vi "Swerve Data Normalize Velocity.vi"(10 "Calcualted Velocities Out":dbl[](array[numeric]), 11 "Swerve Data Out in":T1 {"Back Right"."Angle" scale format="%.3f"; "Back Right"."Velocity" scale=-1.0..1.0 scale format="%.1f"; "Back Left"."Angle" scale format="%.3f"; "Back Left"."Velocity" scale=-1.0..1.0 scale format="%.1f"; "Front Left"."Angle" scale format="%.3f"; "Front Left"."Velocity" scale=-1.0..1.0 scale format="%.1f"; "Front Right"."Angle" scale format="%.3f"; "Front Right"."Velocity" scale=-1.0..1.0 scale format="%.1f"}) -> (3 "Swerve Data Out out":T1 {"Back Right"."Angle" scale format="%.3f"; "Back Right"."Velocity" scale=-1.0..1.0 scale format="%.1f"; "Back Left"."Angle" scale format="%.3f"; "Back Left"."Velocity" scale=-1.0..1.0 scale format="%.1f"; "Front Left"."Angle" scale format="%.3f"; "Front Left"."Velocity" scale=-1.0..1.0 scale format="%.1f"; "Front Right"."Angle" scale format="%.3f"; "Front Right"."Velocity" scale=-1.0..1.0 scale format="%.1f"})   [LabVIEW 2023, in "TShirtWork-SwerveDrive_ACT_ts.lvlib"]
uses:
  TShirtWork-SwerveDrive_ACT_ts.lvlib
  Shared Code/TypeDefs/Cluster_Swerve 4 Steer and Velocity.ctl
  Shared Code/TypeDefs/Cluster_Module Velocity-Direction-Rotations.ctl
  Shared Code/TypeDefs/Level_Velocity plus-minus 1.ctl
  Shared Code/TypeDefs/Dial_Compase heading unit circle CCW positive.ctl
panel:
  # "\"Front\" of Robot"
  # "Right Hand Rule"
  # "X"
  # "+CCW"
  # "Y"
  # "(0,0)"
  # "\"Front\" of Robot"
  # "Right Hand Rule"
  # "X"
  # "+CCW"
  # "Y"
  # "(0,0)"
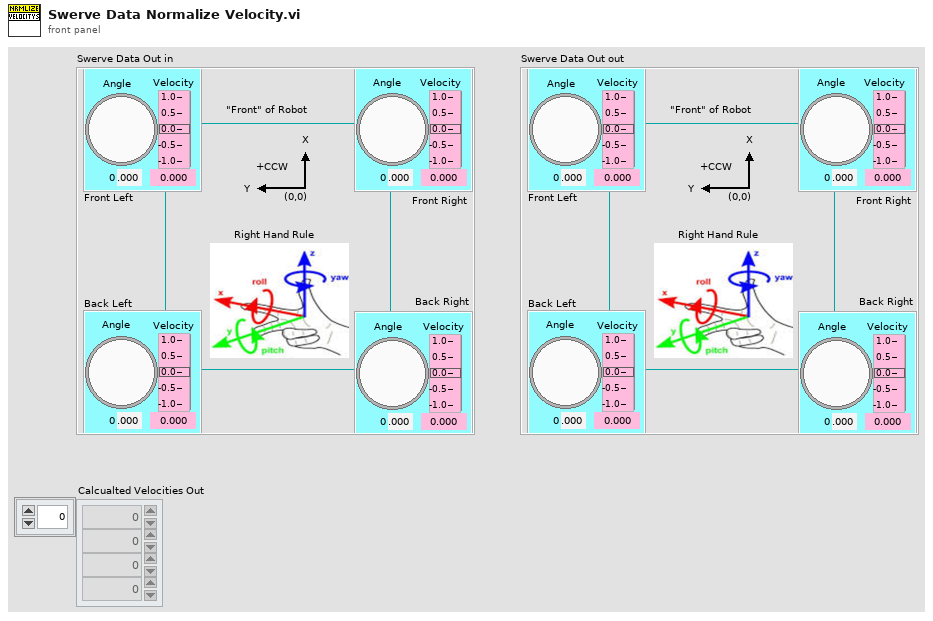
[diagram p1: front panel]
types:
  T1 = typedef "Cluster_Swerve 4 Steer and Velocity.ctl" = cluster{"Front Right":T2, "Front Left":T2, "Back Left":T2, "Back Right":T2}
  T2 = typedef "Cluster_Module Velocity-Direction-Rotations.ctl" = cluster{"Velocity":T3, "Angle":T4, "Rotations Count":dbl}
  T3 = typedef "Level_Velocity plus-minus 1.ctl" = dbl
  T4 = typedef "Dial_Compase heading unit circle CCW positive.ctl" = dbl
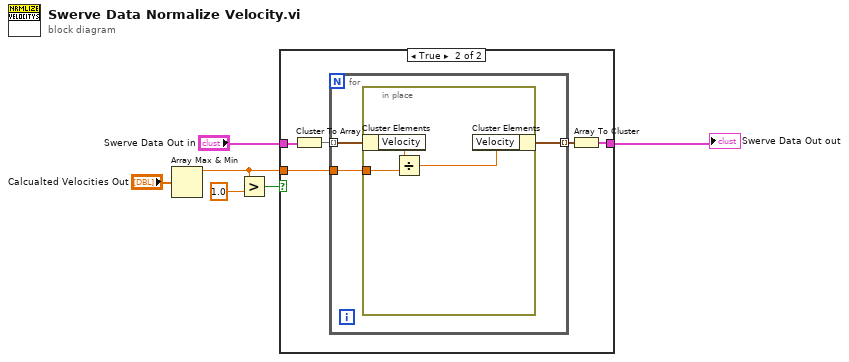
[diagram p0: block diagram]
diagram:
  n1 = Array Max & Min(array="Calcualted Velocities Out") -> (max value=w3:dbl)  [unwired: 3 out]
  n2 = Greater?(x=w3, y=1.0) -> (0:w2:bool)
  n3 = case shown="True" w2 {
    tunnel: "Swerve Data Out in" -> [w7 w12]
    tunnel: [w7 w9] -> w6
    tunnel: w3 -> [_ w8]
    frame False {
    }
    frame True {
      n4 = Cluster To Array(cluster=w12) -> (array=w11:T2[])
      n5 = for {
        tunnel: w11 -> [w15] mode=indexing
        tunnel: [w14] -> w10 mode=indexing
        tunnel: w8 -> [w13]
        n6 = in-place {
          in-place-border: w13 -> [w18]
          n7 = in-place-cluster #1(w15) -> ("Velocity"=w17:T3)
          n8 = Divide(x=w17, y=w18) -> (x/y=w16:T3)
          n9 = in-place-cluster #1("Velocity"=w16) -> (w14:T2)
        }
      }
      n10 = Array To Cluster(array=w10) -> (cluster=w9:cluster{"[0]":T2, "[1]":T2, "[2]":T2, "[3]":T2})
    }
  }
  "Swerve Data Out out" <- w6
